vi "AODO-Initialize DO Clock Source.vi"(0 "Sync Task":refnum<k21>, 5 "DAQmx Device Name":tag="PXI1Slot4", 7 "Fs (Hz)":dbl, 11 "error in (no error)":errorcluster) -> (4 "clock task":refnum<k21>, 15 "error out":errorcluster)   [LabVIEW 2020]
uses:
  <vilib>/DAQmx/create/channels.llb/DAQmx Create Channel (CO-Pulse Generation-Ticks).vi
  <vilib>/DAQmx/configure/timing.llb/DAQmx Timing (Implicit).vi
  <vilib>/DAQmx/configure/trigger.llb/DAQmx Start Trigger (Digital Edge).vi
  <resource>/objmgr/daqmx.rc
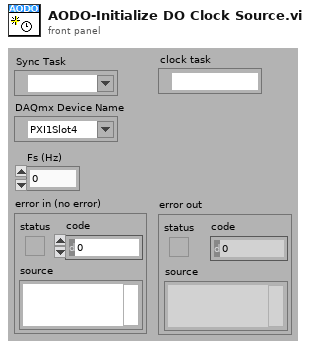
[diagram p1: front panel]
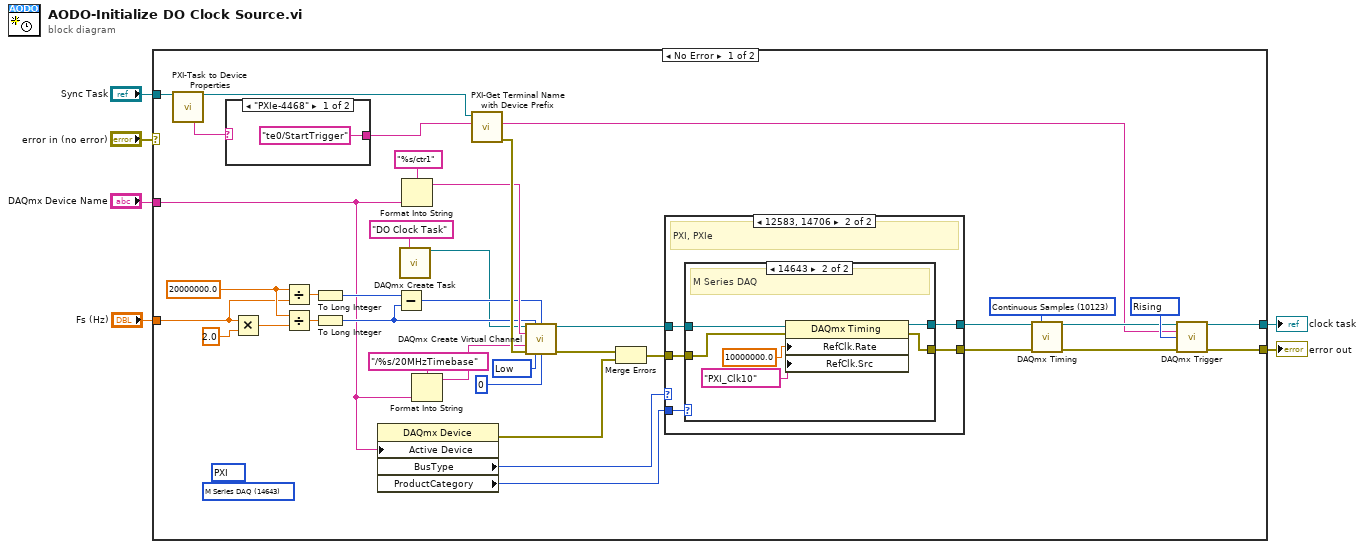
[diagram p0: block diagram]
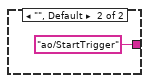
[diagram p2: hidden frame]
diagram:
  n1 = case shown="No Error" "error in (no error)" {
    selector: "error in (no error)" -> [_ w62]
    tunnel: [w44 w62] -> w6
    tunnel: "DAQmx Device Name" -> [w20 _]
    tunnel: "Sync Task" -> [w10 _]
    tunnel: "Fs (Hz)" -> [w16 _]
    tunnel: [w19 _] -> w1
    frame No Error {
      (unwired) 14643 items=["M Series DAQ"=14643, "X Series DAQ"=15858, "E Series DAQ"=14642, "S Series DAQ"=14644, "B Series DAQ"=14662, "SC Series DAQ"=14645, "USB DAQ"=14646, "AO Series"=14647, "Digital I/O"=14648, "TIO Series"=14661, "Dynamic Signal Acquisition"=14649, "Switches"=14650, "CompactDAQ Chassis"=14658, "C Series Module"=14659, "SCXI Module"=14660, "SCC Connector Block"=14704, "SCC Module"=14705, "NI ELVIS"=14755, "Network DAQ"=14829, "SC Express"=15886, "Unknown"=12588] ("ProductCategory")
      (unwired) 12583 items=["PCI"=12582, "PCIe"=13612, "PXI"=12583, "PXIe"=14706, "SCXI"=12584, "SCC"=14707, "PCCard"=12585, "USB"=12586, "CompactDAQ"=14637, "TCP/IP"=14828, "Unknown"=12588, "SwitchBlock"=15870] ("BusType")
      w18 = 20000000.0 ("x")
      w29 = 10214 items=["High"=10192, "Low"=10214] ("idle state")
      w42 = 10280 items=["Rising"=10280, "Falling"=10171] ("Trigger Edge")
      w43 = 10123 items=["Finite Samples"=10178, "Continuous Samples"=10123] ("sample mode")
      n2 = call "PXI-Task to Device Properties.vi"("Task in"=w10) -> ("Task out"=w9:refnum<k21>, "ProductType"=w8:string)  [unwired: 9 in, 4 out]
      n3 = case shown="\"PXIe-4468\"" w8 {
        tunnel: ["te0/StartTrigger" "ao/StartTrigger" ("Local Terminal Name")] -> w7
        frame "PXIe-4468" {
        }
        frame "", Default {
        }
      }
      n4 = Multiply(x=w16, y=2.0 ("x")) -> (x*y=w17:dbl)
      n5 = Divide(x=w18, y=w16) -> (x/y=w27:dbl)
      n6 = Divide(x=w18, y=w17) -> (x/y=w28:dbl)
      n7 = To Long Integer(number=w27) -> (32bit integer=w25:i32)
      n8 = To Long Integer(number=w28) -> (32bit integer=w26:i32)
      n9 = property class="DAQmx Device"("Active Device"=w20) -> (error out=w11:errorcluster, "BusType"=w22:i32, "ProductCategory"=w21:i32)  [unwired: 2 in, 1 out]
      n10 = Subtract(x=w25, y=w26) -> (x-y=w24:i32)
      n11 = call <vilib>:"DAQmx Create Task.vi"("new task name"="DO Clock Task" ("name to assign")) -> ("task out"=w13:refnum<k21>)  [unwired: 13 in, 1 out]
      n12 = Format Into String(format string="%s/ctr1", w20) -> (resulting string=w31:string)  [unwired: 2 in, 1 out]
      n13 = Format Into String(format string="/%s/20MHzTimebase", w20) -> (resulting string=w23:string)  [unwired: 2 in, 1 out]
      n14 = call "PXI-Get Terminal Name with Device Prefix.vi"("Local Terminal Name"=w7, "task/channels in"=w9) -> ("error out"=w36:errorcluster, "Terminal Name with Device Prefix"=w37:string)  [unwired: 7 in, 1 out]
      n15 = call-poly <vilib>:"DAQmx Create Virtual Channel.vi"("task in"=w13, "high ticks"=w26, "low ticks"=w24, "counter"=w31, "source of ticks"=w23, "error in"=w36, "idle state"=w29, "initial delay"=u32 0) -> ("task out"=w34:refnum<k21>, "error out"=w35:errorcluster)  [unwired: 6 in]
      n16 = Merge Errors(w35, w11) -> (w12:errorcluster)
      n17 = case shown="12583, 14706" w22 {
        tunnel: [w48 w53] -> w41
        tunnel: [w47 w52] -> w40
        tunnel: w12 -> [w47 w51]
        tunnel: w34 -> [w48 w50]
        tunnel: w21 -> [_ w49]
        frame 0, Default {
          # "including USB"
        }
        frame 12583, 14706 {
          # "PXI, PXIe"
          n18 = case shown="14643" w49 {
            tunnel: [w55 w61] -> w53
            tunnel: [w54 w60] -> w52
            tunnel: w51 -> [w54 w59]
            tunnel: w50 -> [w55 w58]
            frame 0, Default {
            }
            frame 14643 {
              # "M Series DAQ"
              n19 = property class="DAQmx Timing"(reference=w58, error in=w59, "RefClk.Rate"=10000000.0, "RefClk.Src"=tag "PXI_Clk10") -> (reference out=w61:refnum<k21>, error out=w60:errorcluster)
            }
          }
        }
      }
      n20 = call-poly <vilib>:"DAQmx Timing.vi"("task/channels in"=w41, "sample mode"=w43, "error in"=w40) -> ("task out"=w39:refnum<k21>, "error out"=w38:errorcluster)  [unwired: 11 in]
      n21 = call-poly <vilib>:"DAQmx Trigger.vi"("task/channels in"=w39, "source"=w37, "edge"=w42, "error in"=w38) -> ("task out"=w19:refnum<k21>, "error out"=w44:errorcluster)  [unwired: 10 in]
    }
    frame Error {
    }
  }
  "error out" <- w6
  "clock task" <- w1
